vi "Image roto-translation top level.vi"(0 "ROI to crop (pixels)":T6={"Xmax"=2147483647, "Ymax"=2147483647, "Xmin"=0, "Ymin"=0}, 1 "Theta range (deg)":T5={"theta max (deg)"=180.0, "theta min (deg)"=-180.0}, 2 "Txy range (pixels)":T2={"Tx max (pix)"=2147483647, "Tx min (pix)"=-2147483648, "Ty max (pix)"=2147483647, "Ty min (pix)"=-2147483648}, 3 "Convergence tolerances":T3={"Tx,y tol (abs pix)"=0.001, "Rotation tol (abs deg)"=0.001, "Scale tol (rel fact)"=0.001}, 4 "Max. iters":i32=15, 5 "Controls":T1={"Auto ROI (for rot.)"=FALSE, "Apply scaling"=FALSE, "Apply rotation"=TRUE, "Apply Tx"=TRUE, "Apply Ty"=TRUE, "Keep proc. img"=FALSE}, 6 "Test image file path":path=path "C:/Users/Paul Nathan/Desktop/Building test pictures/Building_pos_9.jpg", 8 "Reference image file path":path=path "C:/Users/Paul Nathan/Desktop/Building test pictures/Building_pos_1.jpg") -> (13 "Converged":bool, 14 "Scale factor":dbl, 15 "Rotation (deg)":dbl, 16 "Tx (pixels)":dbl, 17 "Ty (pixels)":dbl, 18 "Processed test img path":path, 19 "Error Out":errorcluster)   [LabVIEW 2015]
uses:
  Typedefs/ROI bounds.ctl
  Typedefs/Theta range.ctl
  Typedefs/Txy range.ctl
  Typedefs/Top level controls.ctl
panel:
  out "Convergence":T4(graph)
  out "Iter":i32
  out "Image out":T7(plugin-control)
  # "Paul Nathan 10/06/2015, \n07/12/2015, 22/03/2016"
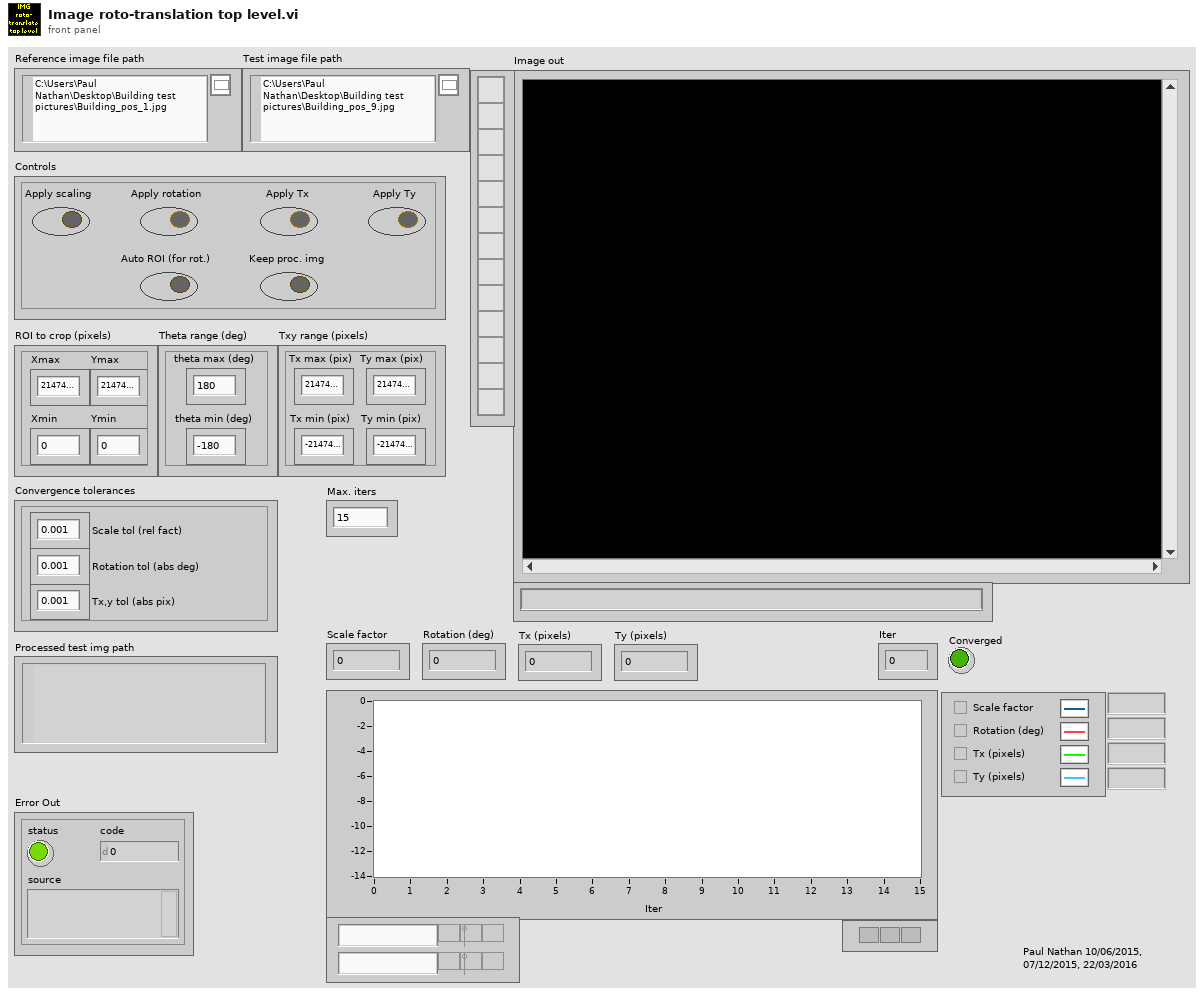
[diagram p1: front panel]
types:
  T1 = typedef "Top level controls.ctl" = cluster{"Auto ROI (for rot.)":bool, "Apply scaling":bool, "Apply rotation":bool, "Apply Tx":bool, "Apply Ty":bool, "Keep proc. img":bool}
  T2 = typedef "Txy range.ctl" = cluster{"Tx max (pix)":i32, "Tx min (pix)":i32, "Ty max (pix)":i32, "Ty min (pix)":i32}
  T3 = cluster{"Tx,y tol (abs pix)":dbl, "Rotation tol (abs deg)":dbl, "Scale tol (rel fact)":dbl}
  T4 = cluster{dbl, dbl, "dx (pix)":dbl, "dy (pix)":dbl}
  T5 = typedef "Theta range.ctl" = cluster{"theta max (deg)":dbl, "theta min (deg)":dbl}
  T6 = typedef "ROI bounds.ctl" = cluster{"Xmax":i32, "Ymax":i32, "Xmin":i32, "Ymin":i32}
  T7 = typedef "IMAQ Image.ctl" = refnum<image>
  T8 = cluster{dbl, dbl, "dx (pix)":dbl, "dy (pix)":dbl}[]
  T9 = typedef "Image Type" = u32
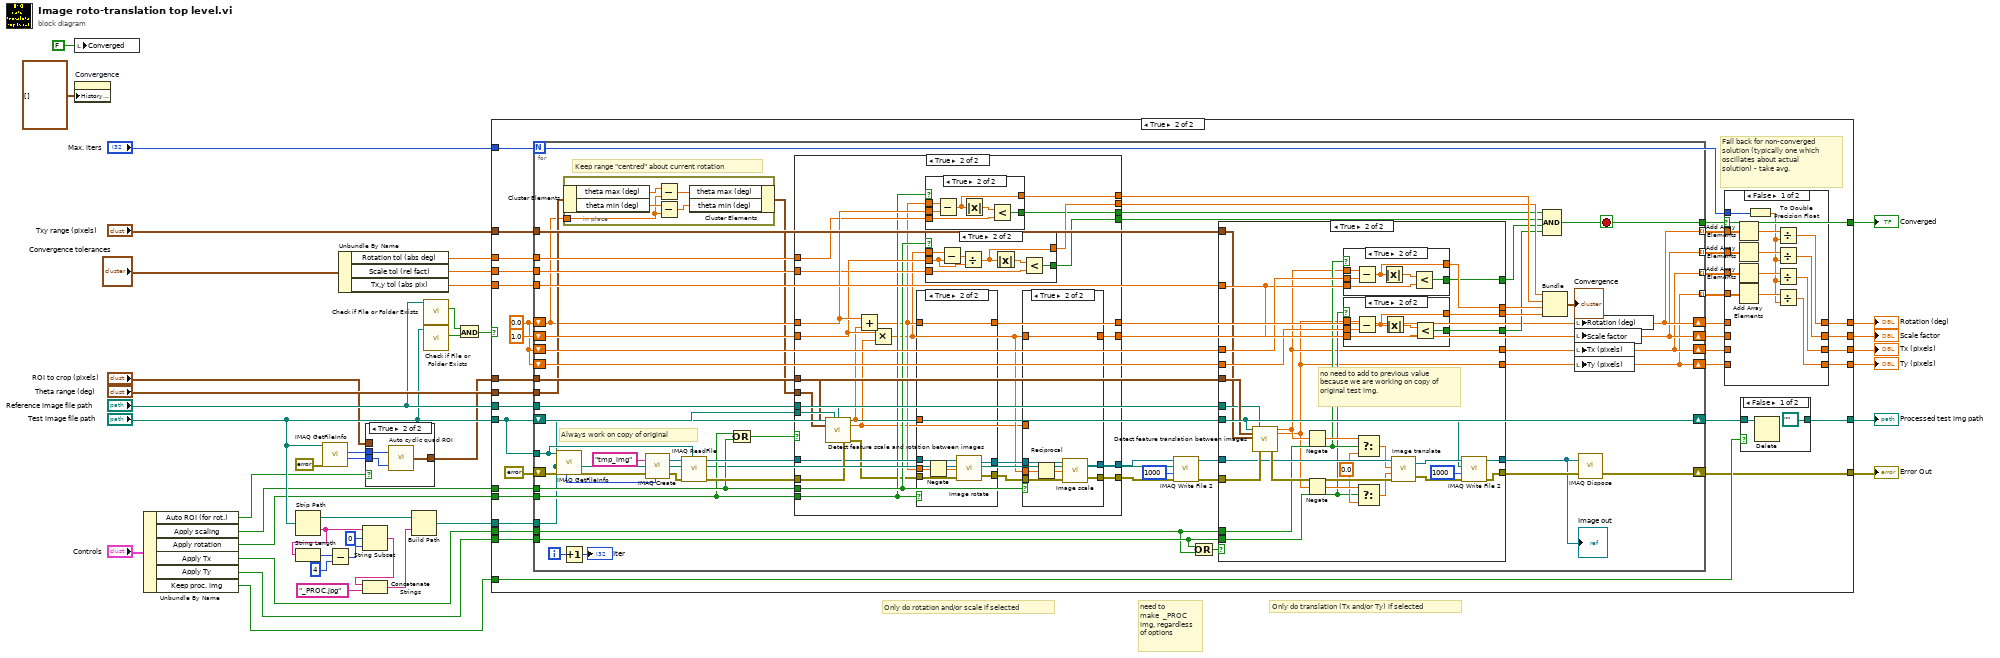
[diagram p0: block diagram]
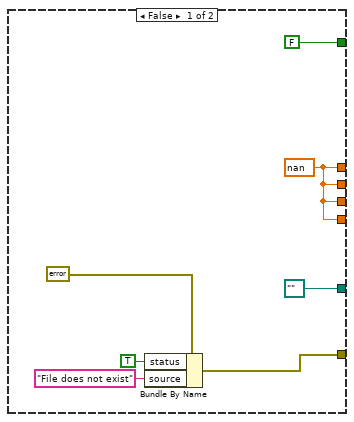
[diagram p3: hidden frame]
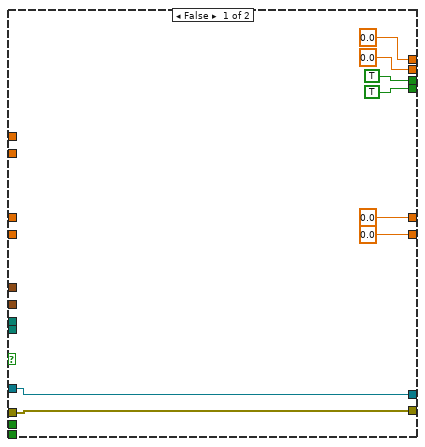
[diagram p5: hidden frame]
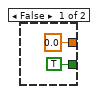
[diagram p6: hidden frame]
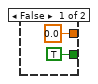
[diagram p7: hidden frame]
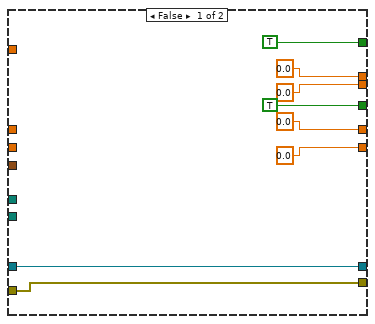
[diagram p10: hidden frame]
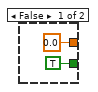
[diagram p11: hidden frame]
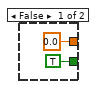
[diagram p12: hidden frame]
diagram:
  # "Only do translation (Tx and/or Ty) if selected"
  # "Only do rotation and/or scale if selected"
  # "need to make  _PROC img, regardless of options"
  n1 = local write "Converged"(FALSE ("Converged")) -> ()
  n2 = property on="Convergence" class="WFChart (strict)"("History Data"=T8 []) -> ()  [unwired: 2 in, 2 out]
  n3 = Unbundle By Name("Controls") -> ("Auto ROI (for rot.)"=w5:bool, "Apply scaling"=w4:bool, "Apply rotation"=w6:bool, "Apply Tx"=w7:bool, "Apply Ty"=w8:bool, "Keep proc. img"=w9:bool)
  n4 = Strip Path(path="Test image file path") -> (stripped path=w35:path, name=w41:string)
  n5 = String Length(string=w41) -> (length=w40:i32)
  n6 = call "IMAQ GetFileInfo"("error in (no error)"=errorcluster {"status"=FALSE, "code"=0, "source"=""}, "File Path"="Test image file path") -> ("Y Resolution"=w17:i32, "X Resolution"=w18:i32)  [unwired: 3 in, 5 out]
  n7 = Subtract(x=w40, y=4) -> (x-y=w34:i32)
  n8 = Unbundle By Name("Convergence tolerances") -> ("Rotation tol (abs deg)"=w13:dbl, "Scale tol (rel fact)"=w12:dbl, "Tx,y tol (abs pix)"=w11:dbl)
  n9 = String Subset(string=w41, offset (0)=0, length (rest)=w34) -> (substring=w38:string)
  n10 = Concatenate Strings(w38, "_PROC.jpg" ("name or relative path")) -> (w36:string)
  n11 = case shown="True" w5 {
    tunnel: [w44 w45] -> w19
    tunnel: w18 -> [_ w47]
    tunnel: w17 -> [_ w46]
    tunnel: "ROI to crop (pixels)" -> [w44 _]
    frame False {
    }
    frame True {
      n12 = call "Auto cyclic quad ROI.vi"("img_H"=w46, "img_W"=w47) -> ("ROI to crop (pixels)"=w45:T6)
    }
  }
  n13 = Build Path(base path=w35, name or relative path=w36) -> (appended path=w42:path)
  n14 = call <vilib>:"Check if File or Folder Exists.vi"("path"="Reference image file path") -> ("file or folder exists?"=w28:bool)  [unwired: 8 in, 2 out]
  n15 = call <vilib>:"Check if File or Folder Exists.vi"("path"="Test image file path") -> ("file or folder exists?"=w29:bool)  [unwired: 8 in, 2 out]
  n16 = And(x=w28, y=w29) -> (x .and. y?=w27:bool)
  n17 = case shown="True" w27 {
    tunnel: "Reference image file path" -> [_ w88]
    tunnel: "Max. iters" -> [_ w64]
    tunnel: w42 -> [_ w87]
    tunnel: [w52 w63] -> w23
    tunnel: [w52 w59] -> w25
    tunnel: "Test image file path" -> [_ w77]
    tunnel: [w52 w61] -> w22
    tunnel: w4 -> [_ w86]
    tunnel: w6 -> [_ w85]
    tunnel: w19 -> [_ w84]
    tunnel: w7 -> [_ w83]
    tunnel: w8 -> [_ w82]
    tunnel: "Theta range (deg)" -> [_ w81]
    tunnel: [path "" ("Test image file path") w78] -> w31
    tunnel: [w50 w76] -> w26
    tunnel: w9 -> [_ w80]
    tunnel: [w52 w57] -> w24
    tunnel: w13 -> [_ w72]
    tunnel: w12 -> [_ w71]
    tunnel: w11 -> [_ w70]
    tunnel: "Txy range (pixels)" -> [_ w69]
    tunnel: [FALSE w55] -> w2
    frame False {
      w52 = nan ("Rotation (deg)")
      n18 = Bundle By Name(cluster=errorcluster {"status"=FALSE, "code"=0, "source"=""} ("error in (no error)"), "status"=TRUE, "source"="File does not exist") -> (w50:errorcluster)
    }
    frame True {
      w73 = 0.0 ("Rotation (deg)")
      # "Fall back for non-converged solution (typically one which oscillates about actual solution) - take avg."
      n19 = for {
        N: w64 -> [_]
        tunnel: w88 -> [w124]
        shift-right: [w120] -> w79
        shift-left: w77 -> [w157]
        tunnel: w87 -> [w120]
        shift-right: [w146] -> w76
        shift-left: errorcluster {"status"=FALSE, "code"=0, "source"=""} ("error in (no error)") -> [w148]
        tunnel: w86 -> [w126]
        tunnel: w85 -> [w125]
        tunnel: w84 -> [w156]
        tunnel: w83 -> [w122]
        tunnel: w82 -> [w123]
        tunnel: w81 -> [w114]
        tunnel: w77 -> [w145]
        shift-right: [w111] -> w62
        shift-left: w73 -> [w113]
        shift-right: [w110] -> w60
        shift-left: 1.0 ("Rotation (deg)") -> [w137]
        shift-right: [w109] -> w58
        shift-left: w73 -> [w134]
        shift-right: [w108] -> w56
        shift-left: w73 -> [w133]
        tunnel: w72 -> [w140]
        tunnel: w71 -> [w128]
        tunnel: w70 -> [w127]
        tunnel: w69 -> [w115]
        tunnel: [w111] -> w68 mode=indexing
        tunnel: [w110] -> w67 mode=indexing
        tunnel: [w109] -> w66 mode=indexing
        tunnel: [w108] -> w65 mode=indexing
        tunnel: [w107] -> w55
        i -> [w159]
        stop <- w107 stop-if-true
        # "Keep range \"centred\" about current rotation"
        # "Always work on copy of original"
        n20 = call "IMAQ GetFileInfo"("error in (no error)"=w148, "File Path"=w145) -> ("error out"=w154:errorcluster, "Image Type"=w155:T9)  [unwired: 3 in, 5 out]
        n21 = Increment(x=w159) -> (x+1=→"Iter":i32)
        n22 = in-place {
          in-place-border: w113 -> [w162]
          n23 = in-place-cluster #1(w114) -> ("theta max (deg)"=w164:dbl, "theta min (deg)"=w163:dbl)
          n24 = Subtract(x=w164, y=w162) -> (x-y=w161:dbl)
          n25 = Subtract(x=w163, y=w162) -> (x-y=w160:dbl)
          n26 = in-place-cluster #1("theta max (deg)"=w161, "theta min (deg)"=w160) -> (w112:T5)
        }
        n27 = call "IMAQ Create"("Image Name"="tmp_img", "Image Type"=w155, "error in (no error)"=w154) -> ("New Image"=w152:T7, "error out"=w153:errorcluster)  [unwired: 2 in]
        n28 = call "IMAQ ReadFile"("File Path"=w145, "error in (no error)"=w153, "Image"=w152) -> ("error out"=w150:errorcluster, "Image Out"=w149:T7)  [unwired: 4 in, 3 out]
        n29 = Or(x=w125, y=w126) -> (x .or. y?=w116:bool)
        n30 = case shown="True" w116 {
          tunnel: w157 -> [_ w199]
          tunnel: w156 -> [_ w198]
          tunnel: w112 -> [_ w197]
          tunnel: w150 -> [w165 w196]
          tunnel: w149 -> [w166 w195]
          tunnel: w113 -> [_ w194]
          tunnel: w140 -> [_ w193]
          tunnel: [0.0 w192] -> w139
          tunnel: [0.0 w191] -> w138
          tunnel: w137 -> [_ w190]
          tunnel: [TRUE w189] -> w132
          tunnel: [TRUE w188] -> w131
          tunnel: w128 -> [_ w187]
          tunnel: [0.0 w174] -> w110
          tunnel: [0.0 w177] -> w111
          tunnel: w126 -> [_ w186]
          tunnel: w125 -> [_ w185]
          tunnel: w124 -> [_ w184]
          tunnel: [w165 w180] -> w118
          tunnel: [w166 w179] -> w117
          frame False {
          }
          frame True {
            n31 = call "Detect feature scale and rotation between images.vi"("ROI to crop (pixels)"=w198, "Test image file path"=w199, "Reference image file path"=w184, "Theta range (deg)"=w197, "Error In"=w196) -> ("Rotation (deg)"=w176:dbl, "Scale factor"=w173:dbl, "Error out"=w183:errorcluster)  [unwired: 6 in, 2 out]
            n32 = Add(x=w194, y=w176) -> (x+y=w178:dbl)
            n33 = Multiply(x=w190, y=w173) -> (x*y=w175:dbl)
            n34 = case shown="True" w185 {
              tunnel: w195 -> [w219 w222]
              tunnel: w183 -> [w218 w226]
              tunnel: w178 -> [_ w223]
              tunnel: [w219 w225] -> w182
              tunnel: [w218 w224] -> w181
              tunnel: w178 -> [_ w220]
              tunnel: [w217 w220] -> w177
              tunnel: w176 -> [w217 _]
              frame False {
              }
              frame True {
                n35 = Negate(x=w223) -> (-x=w221:dbl)
                n36 = call "Image rotate.vi"("Error in"=w226, "Rotation angle, ccw+ (deg)"=w221, "Image in"=w222) -> ("Error Out"=w224:errorcluster, "Image Out"=w225:T7)
              }
            }
            n37 = case shown="True" w185 {
              tunnel: w194 -> [_ w216]
              tunnel: w193 -> [_ w215]
              tunnel: [0.0 w213] -> w192
              tunnel: [TRUE w212] -> w189
              tunnel: w178 -> [_ w211]
              frame False {
              }
              frame True {
                n38 = Subtract(x=w211, y=w216) -> (x-y=w213:dbl)
                n39 = Absolute Value(x=w213) -> (abs(x)=w214:dbl)
                n40 = Less?(x=w214, y=w215) -> (x < y?=w212:bool)
              }
            }
            n41 = case shown="True" w186 {
              tunnel: [0.0 w207] -> w191
              tunnel: w190 -> [_ w205]
              tunnel: [TRUE w204] -> w188
              tunnel: w187 -> [_ w203]
              tunnel: w175 -> [_ w202]
              frame False {
              }
              frame True {
                n42 = Subtract(x=w202, y=w205) -> (x-y=w208:dbl)
                n43 = Divide(x=w208, y=w205) -> (x/y=w207:dbl)
                n44 = Absolute Value(x=w207) -> (abs(x)=w206:dbl)
                n45 = Less?(x=w206, y=w203) -> (x < y?=w204:bool)
              }
            }
            n46 = case shown="True" w186 {
              tunnel: w182 -> [w229 w236]
              tunnel: [w229 w235] -> w179
              tunnel: w181 -> [w228 w234]
              tunnel: [w228 w233] -> w180
              tunnel: w175 -> [_ w232]
              tunnel: w175 -> [_ w230]
              tunnel: [w227 w230] -> w174
              tunnel: w173 -> [w227 _]
              frame False {
              }
              frame True {
                n47 = Reciprocal(x=w232) -> (1/x=w231:dbl)
                n48 = call "Image scale.vi"("Error in"=w234, "Scale factor"=w231, "Image in"=w236) -> ("Error Out"=w233:errorcluster, "Image Out"=w235:T7)
              }
            }
          }
        }
        n49 = call-poly "IMAQ Write File 2"("error in (no error)"=w118, "Image Quality"=u32 1000, "File Path"=w120, "Image"=w117) -> ("error out"=w144:errorcluster, "Image Out (duplicate)"=w143:T7)  [unwired: 6 in]
        n50 = Or(x=w123, y=w122) -> (x .or. y?=w121:bool)
        n51 = case shown="True" w121 {
          tunnel: w156 -> [_ w267]
          tunnel: [w237 w266] -> w147
          tunnel: w144 -> [w237 w264]
          tunnel: w143 -> [w238 w263]
          tunnel: [w238 w262] -> w142
          tunnel: [0.0 w261] -> w136
          tunnel: [0.0 w260] -> w135
          tunnel: w134 -> [_ w259]
          tunnel: w133 -> [_ w258]
          tunnel: w122 -> [_ w250]
          tunnel: w123 -> [_ w249]
          tunnel: [TRUE ("f") w251] -> w130
          tunnel: [TRUE ("f") w248] -> w129
          tunnel: w127 -> [_ w257]
          tunnel: [0.0 ("dy (pix)") w246] -> w108
          tunnel: [0.0 ("dx (pix)") w247] -> w109
          tunnel: w124 -> [_ w256]
          tunnel: w120 -> [_ w255]
          tunnel: w115 -> [_ w245]
          frame False {
          }
          frame True {
            w252 = 0.0 ("f")
            # "no need to add to previous value because we are working on copy of original test img."
            n52 = call "Detect feature translation between images.vi"("Test image file path"=w255, "ROI to crop (pixels)"=w267, "Txy range (pixels)"=w245, "Reference image file path"=w256, "Error In"=w264) -> ("Error out"=w265:errorcluster, "dx (pix)"=w247:dbl, "dy (pix)"=w246:dbl)  [unwired: 10 in, 2 out]
            n53 = Negate(x=w247) -> (-x=w269:dbl)
            n54 = Negate(x=w246) -> (-x=w268:dbl)
            n55 = case shown="True" w250 {
              tunnel: [0.0 w288] -> w261
              tunnel: w259 -> [_ w286]
              tunnel: w257 -> [_ w285]
              tunnel: w247 -> [_ w284]
              tunnel: [TRUE w283] -> w251
              frame False {
              }
              frame True {
                n56 = Subtract(x=w284, y=w286) -> (x-y=w288:dbl)
                n57 = Absolute Value(x=w288) -> (abs(x)=w287:dbl)
                n58 = Less?(x=w287, y=w285) -> (x < y?=w283:bool)
              }
            }
            n59 = case shown="True" w249 {
              tunnel: [0.0 w280] -> w260
              tunnel: w258 -> [_ w278]
              tunnel: w257 -> [_ w277]
              tunnel: w246 -> [_ w276]
              tunnel: [TRUE w275] -> w248
              frame False {
              }
              frame True {
                n60 = Subtract(x=w276, y=w278) -> (x-y=w280:dbl)
                n61 = Absolute Value(x=w280) -> (abs(x)=w279:dbl)
                n62 = Less?(x=w279, y=w277) -> (x < y?=w275:bool)
              }
            }
            n63 = Select(t=w269, s=w250, f=w252) -> (s? t:f=w254:dbl)
            n64 = Select(t=w268, s=w249, f=w252) -> (s? t:f=w253:dbl)
            n65 = call "Image translate.vi"("Error in"=w265, "Ty (pix)"=w253, "Tx (pix)"=w254, "Image in"=w263) -> ("Error Out"=w270:errorcluster, "Image Out"=w271:T7)
            n66 = call-poly "IMAQ Write File 2"("error in (no error)"=w270, "Image Quality"=u32 1000, "File Path"=w255, "Image"=w271) -> ("error out"=w266:errorcluster, "Image Out (duplicate)"=w262:T7)  [unwired: 6 in]
          }
        }
        "Image out" <- w142
        n67 = Compound Arithmetic op=AND(w132, w131, w130, w129) -> (w107:bool)
        n68 = Bundle(w138, w139, w136, w135) -> (→"Convergence":cluster{dbl, dbl, dbl, dbl})  [unwired: 1 in]
        n69 = local write "Rotation (deg)"(w111) -> ()
        n70 = local write "Scale factor"(w110) -> ()
        n71 = local write "Tx (pixels)"(w109) -> ()
        n72 = local write "Ty (pixels)"(w108) -> ()
        n73 = call "IMAQ Dispose"("Image"=w142, "error in (no error)"=w147) -> ("error out"=w146:errorcluster)  [unwired: 4 in]
      }
      n74 = case shown="False" w55 {
        tunnel: w68 -> [w102 _]
        tunnel: w67 -> [w101 _]
        tunnel: w66 -> [w100 _]
        tunnel: w65 -> [w99 _]
        tunnel: w64 -> [w94 _]
        tunnel: [w90 w106] -> w63
        tunnel: w62 -> [_ w106]
        tunnel: [w91 w105] -> w61
        tunnel: w60 -> [_ w105]
        tunnel: [w92 w104] -> w59
        tunnel: w58 -> [_ w104]
        tunnel: [w93 w103] -> w57
        tunnel: w56 -> [_ w103]
        frame False {
          n75 = Add Array Elements(numeric array=w102) -> (sum=w98:dbl)
          n76 = Add Array Elements(numeric array=w101) -> (sum=w97:dbl)
          n77 = Add Array Elements(numeric array=w100) -> (sum=w96:dbl)
          n78 = Add Array Elements(numeric array=w99) -> (sum=w95:dbl)
          n79 = To Double Precision Float(number=w94) -> (double precision float=w89:dbl)
          n80 = Divide(x=w98, y=w89) -> (x/y=w90:dbl)
          n81 = Divide(x=w97, y=w89) -> (x/y=w91:dbl)
          n82 = Divide(x=w96, y=w89) -> (x/y=w92:dbl)
          n83 = Divide(x=w95, y=w89) -> (x/y=w93:dbl)
        }
        frame True {
        }
      }
      n84 = case shown="False" w80 {
        tunnel: w79 -> [w289 w291]
        tunnel: [path "" ("Test image file path") w291] -> w78
        frame False {
          n85 = Delete(path (use dialog)=w289) -> ()  [unwired: 4 in, 3 out]
        }
        frame True {
        }
      }
    }
  }
  "Processed test img path" <- w31
  "Error Out" <- w26
  "Tx (pixels)" <- w25
  "Ty (pixels)" <- w24
  "Rotation (deg)" <- w23
  "Scale factor" <- w22
  "Converged" <- w2
